vi "ApplicationSetup_Read.vi"(8 "error in (no error)":errorcluster, 10 "Path":path, 11 "OXYGEN Ref In":refnum<visa-resource-name>) -> (0 "error out":errorcluster, 1 "communication_data":T1, 2 "Setup XML-String":string, 3 "OXYGEN Ref Out":refnum<visa-resource-name>)   [LabVIEW 2018, in "OXYGEN.lvlib"]
doc: "Download the current measurement setup or, if a path is specified, the measurement setup referenced to path from the device."
uses:
  OXYGEN.lvlib
  TypeDefs/Cluster_RawCommData.ctl
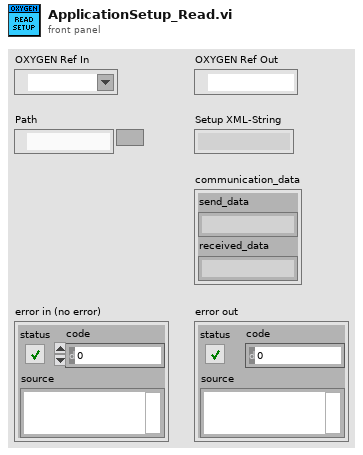
[diagram p1: front panel]
types:
  T1 = typedef "OXYGEN.lvlib/Cluster_RawCommData.ctl" = cluster{"send_data":string, "received_data":string}
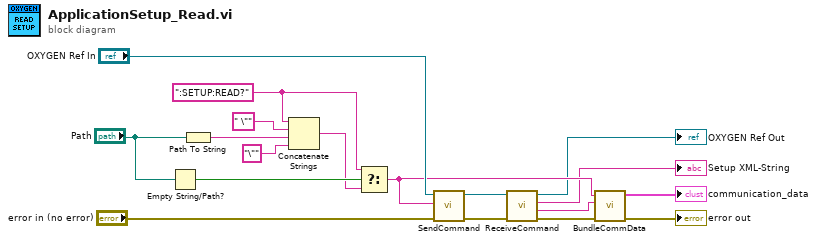
[diagram p0: block diagram]
diagram:
  w7 = ":SETUP:READ?"
  n1 = Empty String/Path?(string/path="Path") -> (empty?=w11:bool)
  n2 = Path To String(path="Path") -> (string=w13:string)
  n3 = Concatenate Strings(w7, " \"", w13, "\"" ("string")) -> (w10:string)
  n4 = Select(t=w7, s=w11, f=w10) -> (s? t:f=w9:string)
  n5 = call "SendCommand.vi"("error in (no error)"="error in (no error)", "String to Send"=w9, "OXY_SCPI Reseource In"="OXYGEN Ref In") -> ("error out"=w6:errorcluster, "OXY_SCPI Reseource Out"=w5:refnum<visa-resource-name>)  [unwired: 7 in]
  n6 = call "ReceiveCommand.vi"("error in (no error)"=w6, "OXY_SCPI Reseource In"=w5) -> ("error out"=w3:errorcluster, "received Data with Header"=w1:string, "received Data"=→"Setup XML-String":string, "OXY_SCPI Reseource Out"=→"OXYGEN Ref Out":refnum<visa-resource-name>)  [unwired: 6 in]
  n7 = call "BundleCommData.vi"("error in (no error)"=w3, "received_data"=w1, "send_data"=w9) -> ("error out"=→"error out":errorcluster, "communication_data"=→"communication_data":T1)  [unwired: 7 in]
